vi "Set Message Metatdata.vi"(6 "Message Type":T1, 8 "error in (no error)":errorcluster, 10 "References":T2) -> (0 "error out":errorcluster)   [LabVIEW 2023, in "Message Maker.lvclass"]
doc: "Writes checksums and message info to the message class's meta data. These checksums are used to detect changes in the source VIs\n\nAuthor: Derek Trepanier\nCopyright: MGI 2015"
uses:
  Message Maker.lvclass
  Scripting Refs.ctl
  Message Type.ctl
  Method Signature.ctl
  <vilib>/LabVIEW Icon API/lv_icon/Classes/Icon/Icon.lvclass
  Message Maker.lvclass/Message Maker.ctl
  <vilib>/LabVIEW Icon API/LabVIEW Icon API.lvlib
panel:
  out "Array":string[](array[string])
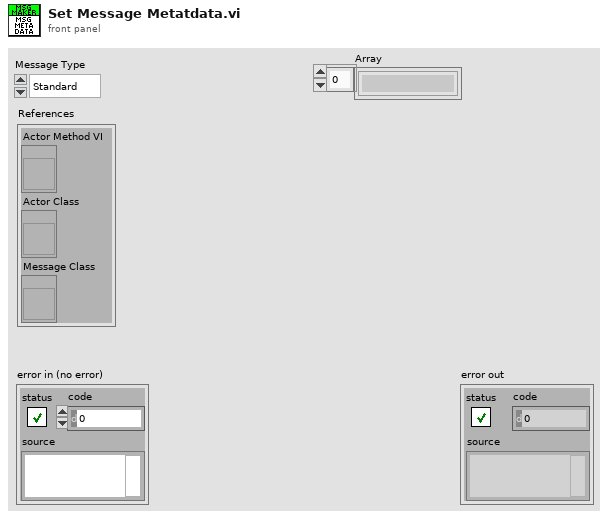
[diagram p1: front panel]
types:
  T1 = typedef "Message Maker.lvclass/Message Type.ctl" = enum16{"Standard", "Async"}
  T2 = typedef "Message Maker.lvclass/Scripting Refs.ctl" = cluster{"Actor Method VI":refnum<vi>, "Actor Class":refnum<vi>, "Message Class":refnum<vi>}
  T3 = typedef "Message Maker.lvclass/Method Signature.ctl" = cluster{"Connector Pane":variant, "Description":string, "Icon":refnum<class "Icon.lvclass">}
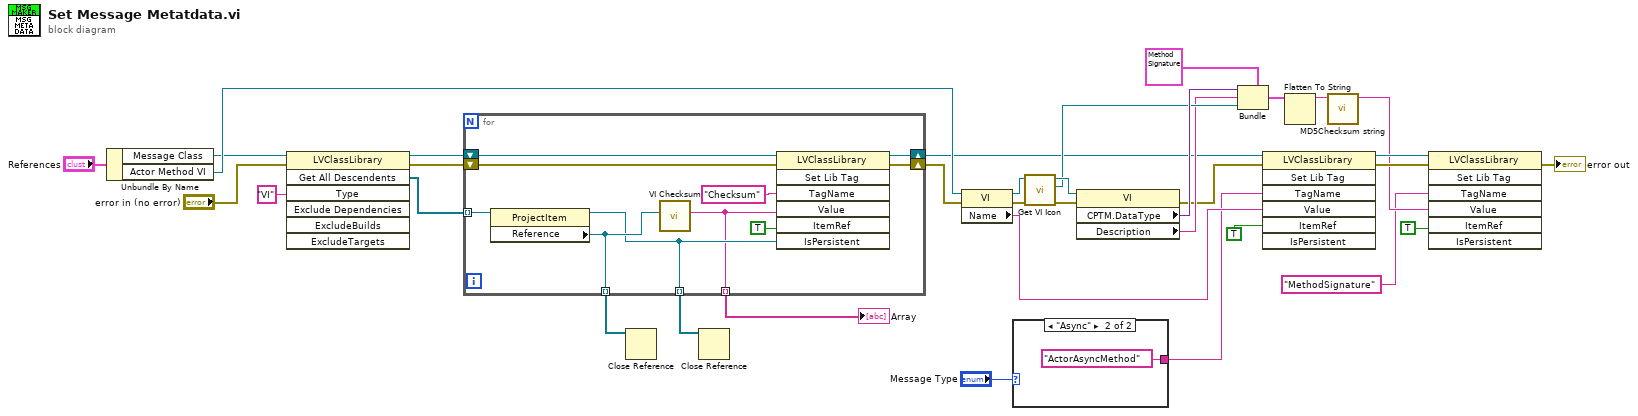
[diagram p0: block diagram]
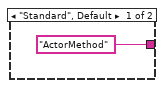
[diagram p2: hidden frame]
diagram:
  n1 = Unbundle By Name("References") -> ("Message Class"=w14:refnum<vi>, "Actor Method VI"=w18:refnum<vi>)
  n2 = invoke class="LVClassLibrary" method="Get All Descendents"(reference=w14, error in="error in (no error)", "Type"="VI") -> (reference out=w10:refnum<vi>, error out=w9:errorcluster, "All Descendents"=w7:refnum<vi>[])  [unwired: 4 in, 4 out]
  n3 = for {
    tunnel: w7 -> [w44] mode=indexing
    shift-right: [w42] -> w13
    shift-left: w10 -> [w43]
    shift-right: [w40] -> w12
    shift-left: w9 -> [w41]
    tunnel: [w37] -> w5 mode=indexing
    tunnel: [w36] -> w6 mode=indexing
    tunnel: [w35] -> w4 mode=indexing
    n4 = property class="ProjectItem"(reference=w44) -> (reference out=w36:refnum<vi>, "Reference"=w37:refnum<vi>)  [unwired: 1 in, 1 out]
    n5 = call "VI Checksum.vi"("VI"=w37) -> ("VI Checksum"=w35:string)  [unwired: 10 in]
    n6 = invoke class="LVClassLibrary" method="Set Lib Tag"(reference=w43, error in=w41, "TagName"="Checksum" ("Tag Name"), "Value"=w35, "ItemRef"=TRUE ("Is Persistent"), "IsPersistent"=w36) -> (reference out=w42:refnum<vi>, error out=w40:errorcluster)  [unwired: 1 in, 5 out]
  }
  "Array" <- w4
  n7 = Close Reference(reference=w5) -> ()  [unwired: 1 in, 1 out]
  n8 = Close Reference(reference=w6) -> ()  [unwired: 1 in, 1 out]
  n9 = property class="VI"(reference=w18, error in=w12) -> (reference out=w29:refnum<vi>, error out=w27:errorcluster, "Name"=w28:string)
  n10 = case shown="\"Async\"" "Message Type" {
    tunnel: ["ActorMethod" ("Tag Name") "ActorAsyncMethod" ("Tag Name")] -> w2
    frame "Standard", Default {
    }
    frame "Async" {
    }
  }
  n11 = call <vilib>:"Get VI Icon.vi"("error in (no error)"=w27, "VI Refnum in"=w29) -> ("error out"=w26:errorcluster, "Icon"=w32:refnum<class "Icon.lvclass">, "VI Refnum out"=w34:refnum<vi>)  [unwired: 7 in]
  n12 = property class="VI"(reference=w34, error in=w26) -> (error out=w25:errorcluster, "CPTM.DataType"=w33:variant, "Description"=w31:string)  [unwired: 1 out]
  n13 = Bundle(cluster=T3 {"Connector Pane"=variant, "Description"="", "Icon"=refnum} ("output cluster"), "Connector Pane"=w33, "Description"=w31, "Icon"=w32) -> (w17:T3)
  n14 = invoke class="LVClassLibrary" method="Set Lib Tag"(reference=w13, error in=w25, "TagName"=w2, "Value"=w28, "ItemRef"=TRUE ("Is Persistent")) -> (reference out=w23:refnum<vi>, error out=w21:errorcluster)  [unwired: 2 in, 5 out]
  n15 = Flatten To String(anything=w17) -> (data string=w16:string)  [unwired: 3 in, 2 out]
  n16 = call <vilib>:"MD5Checksum string.vi"("Message String"=w16) -> ("MD5 message-digest"=w15:string)  [unwired: 10 in]
  n17 = invoke class="LVClassLibrary" method="Set Lib Tag"(reference=w23, error in=w21, "TagName"="MethodSignature" ("Tag Name"), "Value"=w15, "ItemRef"=TRUE ("Is Persistent")) -> (error out=→"error out":errorcluster)  [unwired: 2 in, 6 out]
